vi "Read Stack Header (SubVI).vi"(11 "File REF In":refnum<file>) -> (0 "Stack Header":T1={"ID Code"=[32, 202, 103, 187], "Stack Header Size"=512, "Stack Size"=9610440, "N Frames"=180}, 3 "File REF Out":refnum<file>)   [LabVIEW 2015]
uses:
  Controls/Stack Header.ctl
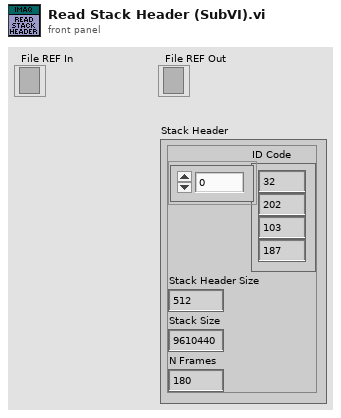
[diagram p1: front panel]
types:
  T1 = typedef "Stack Header.ctl" = cluster{"ID Code":u8[], "Stack Header Size":i32, "Stack Size":i32, "N Frames":i32}
  T2 = enum16{"big-endian, network order", "native, host order", "little-endian"}
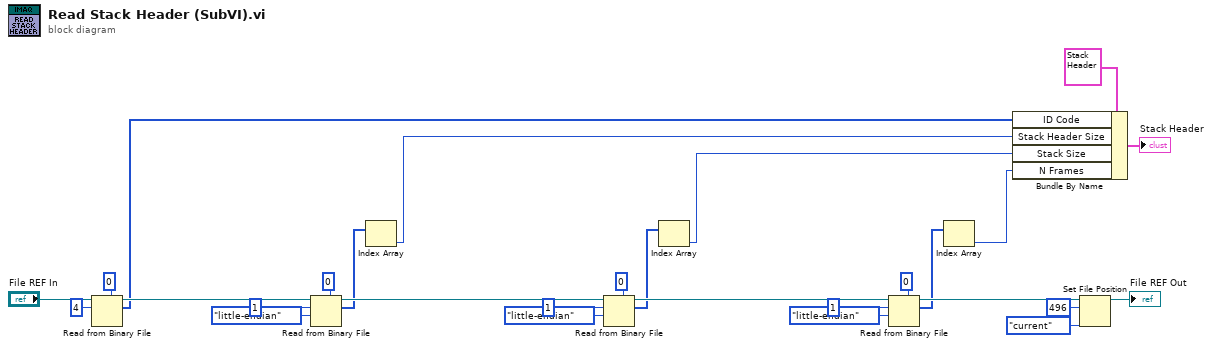
[diagram p0: block diagram]
diagram:
  n1 = Read from Binary File(5:u8 0, 10:4 ("count (1)"), 11:"File REF In") -> (2:w6:u8[], 3:w11:refnum<file>)  [unwired: 3 in, 2 out]
  n2 = Read from Binary File(5:0, 9:T2."little-endian" ("byte order (0:big-endian, network order)"), 10:1 ("count (1)"), 11:w11) -> (2:w13:i32[], 3:w19:refnum<file>)  [unwired: 2 in, 2 out]
  n3 = Index Array(array=w13) -> (element=w5:i32)  [unwired: 1 in]
  n4 = Read from Binary File(5:0, 9:T2."little-endian" ("byte order (0:big-endian, network order)"), 10:1 ("count (1)"), 11:w19) -> (2:w16:i32[], 3:w24:refnum<file>)  [unwired: 2 in, 2 out]
  n5 = Index Array(array=w16) -> (element=w4:i32)  [unwired: 1 in]
  n6 = Read from Binary File(5:0, 9:T2."little-endian" ("byte order (0:big-endian, network order)"), 10:1 ("count (1)"), 11:w24) -> (2:w22:i32[], 3:w25:refnum<file>)  [unwired: 2 in, 2 out]
  n7 = Index Array(array=w22) -> (element=w3:i32)  [unwired: 1 in]
  n8 = Bundle By Name(cluster=T1 {"ID Code"=[32, 202, 103, 187], "Stack Header Size"=512, "Stack Size"=9610440, "N Frames"=180}, "ID Code"=w6, "Stack Header Size"=w5, "Stack Size"=w4, "N Frames"=w3) -> (→"Stack Header":T1)
  n9 = Set File Position(offset (in bytes) (0)=i64 496, refnum=w25, from (0:start)=enum16{"start", "end", "current"}."current") -> (refnum out=→"File REF Out":refnum<file>)  [unwired: 1 in, 1 out]
